vi "Raw to g.vi"(11 "Input":i16) -> (3 "Output":dbl)   [LabVIEW 2015]
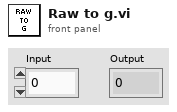
[diagram p1: front panel]
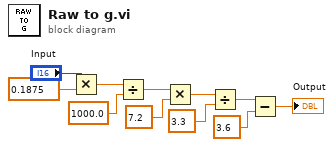
[diagram p0: block diagram]
diagram:
  n1 = Multiply(x="Input", y=0.1875) -> (x*y=w2:dbl)
  n2 = Divide(x=w2, y=1000.0) -> (x/y=w4:dbl)
  n3 = Multiply(x=w4, y=7.2) -> (x*y=w6:dbl)
  n4 = Divide(x=w6, y=3.3) -> (x/y=w8:dbl)
  n5 = Subtract(x=w8, y=3.6) -> (x-y=→"Output":dbl)
